vi "DT3120_NewDevice.vi"(8 "error in (no error)":errorcluster, 11 "Alias":string) -> (0 "error out":errorcluster, 1 "Frame Info":T1, 2 "CurDevCaps":T2, 3 "DevId":i32)   [LabVIEW 2013]
uses:
  olimg32.dll
  olfg32.dll
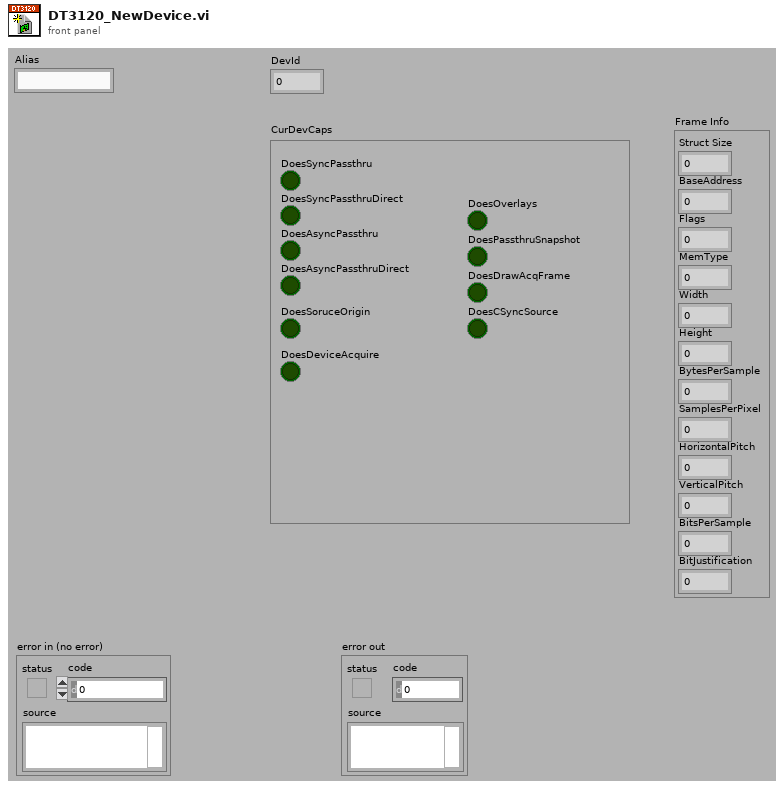
[diagram p1: front panel]
types:
  T1 = cluster{"Struct Size":u32, "BaseAddress":u32, "Flags":u32, "MemType":u32, "Width":u16, "Height":u16, "BytesPerSample":u16, "SamplesPerPixel":u16, "HorizontalPitch":u16, "VerticalPitch":u16, "BitsPerSample":u16, "BitJustification":u32}
  T2 = cluster{"DoesSyncPassthru":bool, "DoesSyncPassthruDirect":bool, "DoesAsyncPassthru":bool, "DoesAsyncPassthruDirect":bool, "DoesSoruceOrigin":bool, "DoesDeviceAcquire":bool, "DoesOverlays":bool, "DoesPassthruSnapshot":bool, "DoesDrawAcqFrame":bool, "DoesCSyncSource":bool}
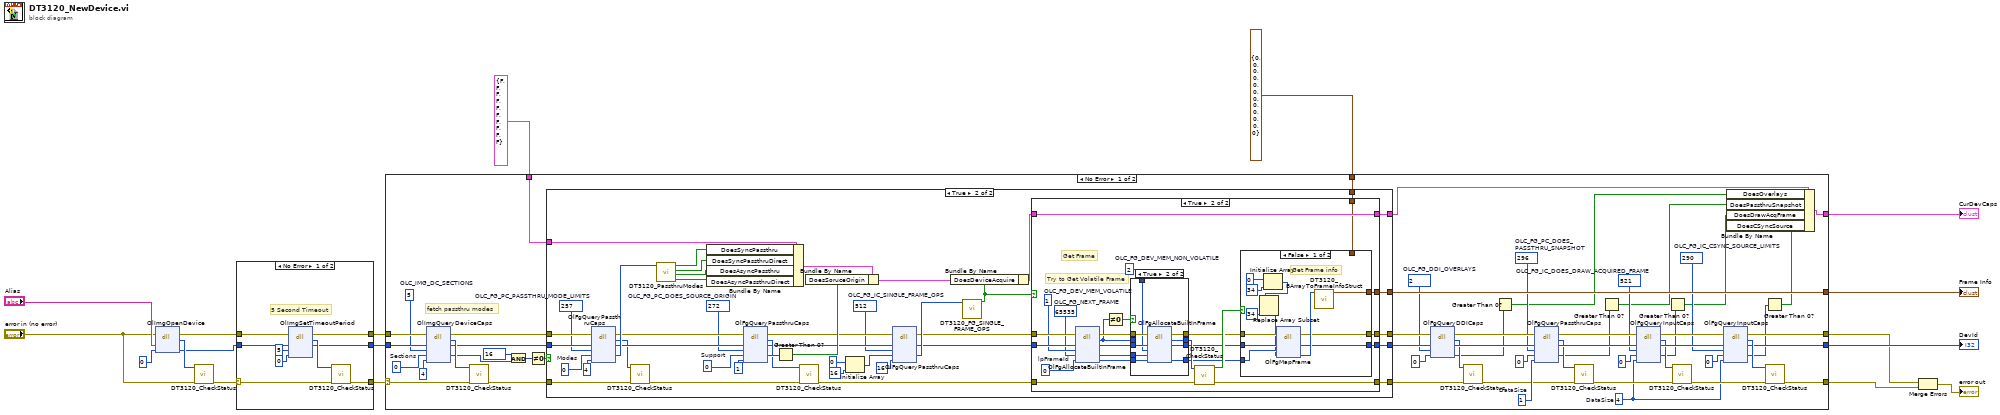
[diagram p0: block diagram]
diagram:
  n1 = dll-call lib="C:/Users/dhaehnel/Documents/Workspace/Labview_Workspace/labviewlib/MT Scan/SubVIs/olimg32.dll" fn="OlImgOpenDevice"(error in="error in (no error)", "Alias"="Alias", "lpDevId"=0 ("DevId")) -> (error out=w14:errorcluster, "Status"=w17:u32, "lpDevId"=w13:i32)  [unwired: 3 in, 1 out]
  n2 = call "DT3120_CheckStatus.vi"("error in"="error in (no error)", "Status"=w17) -> ("error out"=w12:errorcluster)  [unwired: 9 out]
  n3 = case shown="No Error" w12 {
    selector: w12 -> [w22 w30]
    tunnel: w14 -> [w27 w29]
    tunnel: w13 -> [w24 w28]
    tunnel: [w21 w29] -> w9
    tunnel: [w20 w30] -> w11
    tunnel: [w19 w28] -> w10
    frame No Error {
      # "5 Second Timeout"
      n4 = dll-call lib="C:/Users/dhaehnel/Documents/Workspace/Labview_Workspace/labviewlib/MT Scan/SubVIs/olimg32.dll" fn="OlImgSetTimeoutPeriod"(error in=w27, "DevId"=w24, "Period"=u32 5, "lpPeriod"=u32 0) -> (error out=w21:errorcluster, "Status"=w23:u32, "DevId"=w19:i32)  [unwired: 3 in, 2 out]
      n5 = call "DT3120_CheckStatus.vi"("error in"=w22, "Status"=w23) -> ("error out"=w20:errorcluster)  [unwired: 9 out]
    }
    frame Error {
    }
  }
  n6 = case shown="No Error" w11 {
    selector: w11 -> [w83 w196]
    tunnel: w9 -> [w86 w195]
    tunnel: w10 -> [w85 w194]
    tunnel: [w43 w195] -> w6
    tunnel: [w44 w196] -> w7
    tunnel: [w42 w194] -> w8
    tunnel: T2 {"DoesSyncPassthru"=FALSE, "DoesSyncPassthruDirect"=FALSE, "DoesAsyncPassthru"=FALSE, "DoesAsyncPassthruDirect"=FALSE, "DoesSoruceOrigin"=FALSE, "DoesDeviceAcquire"=FALSE, "DoesOverlays"=FALSE, "DoesPassthruSnapshot"=FALSE, "DoesDrawAcqFrame"=FALSE, "DoesCSyncSource"=FALSE} ("CurDevCaps") -> [w72 w193]
    tunnel: [w32 w193] -> w1
    tunnel: [w71 w192] -> w4
    tunnel: T1 {"Struct Size"=0, "BaseAddress"=0, "Flags"=0, "MemType"=0, "Width"=0, "Height"=0, "BytesPerSample"=0, "SamplesPerPixel"=0, "HorizontalPitch"=0, "VerticalPitch"=0, "BitsPerSample"=0, "BitJustification"=0} ("Frame Info") -> [w70 w192]
    frame No Error {
      w31 = u32 4  # DataSize
      w53 = 290  # OLC_FG_IC_CSYNC_SOURCE_LIMITS
      w60 = 521  # OLC_FG_IC_DOES_DRAW_ACQUIRED_FRAME
      w55 = u32 1  # DataSize
      w61 = 296  # OLC_FG_PC_DOES_PASSTHRU_SNAPSHOT
      w67 = 2  # OLC_FG_DDI_OVERLAYS
      w81 = u32 0  # Sections
      w82 = 5  # OLC_IMG_DC_SECTIONS
      # "fetch passthru modes"
      n7 = dll-call lib="C:/Users/dhaehnel/Documents/Workspace/Labview_Workspace/labviewlib/MT Scan/SubVIs/olimg32.dll" fn="OlImgQueryDeviceCaps"(error in=w86, "DevId"=w85, "Key"=w82, "lpData"=w81, "DataSize"=u32 4) -> (error out=w76:errorcluster, "Status"=w84:u32, "DevId"=w75:i32, "lpData"=w79:u32)  [unwired: 4 in, 1 out]
      n8 = call "DT3120_CheckStatus.vi"("error in"=w83, "Status"=w84) -> ("error out"=w74:errorcluster)  [unwired: 9 out]
      n9 = And(x=u32 16, y=w79) -> (x .and. y?=w77:u32)
      n10 = Not Equal To 0?(x=w77) -> (x != 0?=w73:bool)
      n11 = case shown="True" w73 {
        tunnel: w76 -> [w91 w134]
        tunnel: w75 -> [w90 w133]
        tunnel: w74 -> [w89 w122]
        tunnel: [w89 w101] -> w52
        tunnel: [w91 w97] -> w69
        tunnel: [w90 w96] -> w68
        tunnel: w72 -> [w88 w113]
        tunnel: [w88 w94] -> w33
        tunnel: [w87 w93] -> w71
        tunnel: w70 -> [w87 w92]
        frame False {
        }
        frame True {
          w125 = u8 0  # Support
          w109 = 512  # OLC_FG_IC_SINGLE_FRAME_OPS
          w126 = 272  # OLC_FG_PC_DOES_SOURCE_ORIGIN
          w131 = u32 0  # Modes
          w132 = 257  # OLC_FG_PC_PASSTHRU_MODE_LIMITS
          n12 = dll-call lib="C:/Users/dhaehnel/Documents/Workspace/Labview_Workspace/labviewlib/MT Scan/SubVIs/olfg32.dll" fn="OlFgQueryPassthruCaps"(error in=w134, "DevId"=w133, "Key"=w132, "lpData"=w131, "DataSize"=u32 4) -> (error out=w128:errorcluster, "Status"=w121:u32, "DevId"=w127:i32, "lpData"=w129:u32)  [unwired: 4 in, 1 out]
          n13 = call "DT3120_CheckStatus.vi"("error in"=w122, "Status"=w121) -> ("error out"=w120:errorcluster)  [unwired: 9 out]
          n14 = call "DT3120_PassthruModes.vi"("Modes"=w129) -> ("DoesAsyncPassthruDirect"=w114:bool, "DoesAsyncPassthru"=w115:bool, "DoesSyncPassthruDirect"=w116:bool, "DoesSyncPassthru"=w117:bool)  [unwired: 7 out]
          n15 = Bundle By Name(cluster=w113, "DoesSyncPassthru"=w117, "DoesSyncPassthruDirect"=w116, "DoesAsyncPassthru"=w115, "DoesAsyncPassthruDirect"=w114) -> (w112:T2)
          n16 = dll-call lib="C:/Users/dhaehnel/Documents/Workspace/Labview_Workspace/labviewlib/MT Scan/SubVIs/olfg32.dll" fn="OlFgQueryPassthruCaps"(error in=w128, "DevId"=w127, "Key"=w126, "lpData"=w125, "DataSize"=u32 1) -> (error out=w110:errorcluster, "Status"=w119:u32, "DevId"=w111:i32, "lpData"=w123:u8)  [unwired: 4 in, 1 out]
          n17 = Greater Than 0?(x=w123) -> (x > 0?=w118:bool)
          n18 = call "DT3120_CheckStatus.vi"("error in"=w120, "Status"=w119) -> ("error out"=w105:errorcluster)  [unwired: 9 out]
          n19 = Bundle By Name(cluster=w112, "DoesSoruceOrigin"=w118) -> (w106:T2)
          n20 = Initialize Array(u8 0, 16 ("dimension size")) -> (w99:u8[])
          n21 = dll-call lib="C:/Users/dhaehnel/Documents/Workspace/Labview_Workspace/labviewlib/MT Scan/SubVIs/olfg32.dll" fn="OlFgQueryPassthruCaps"(error in=w110, "DevId"=w111, "Key"=w109, "lpData"=w99, "DataSize"=u32 16) -> (error out=w103:errorcluster, "DevId"=w102:i32, "lpData"=w107:u8[])  [unwired: 4 in, 2 out]
          n22 = call "DT3120_FG_SINGLE_FRAME_OPS.vi"("OLT_FG_SINGLE_FRAME_OPS"=w107) -> ("DoesSyncPassthru"=w104:bool)  [unwired: 10 out]
          n23 = Bundle By Name(cluster=w106, "DoesDeviceAcquire"=w104) -> (w95:T2)
          n24 = case shown="True" w104 {
            tunnel: w105 -> [w139 w151]
            tunnel: w103 -> [w138 w163]
            tunnel: w102 -> [w137 w162]
            tunnel: [w139 w149] -> w101
            tunnel: [w138 w144] -> w97
            tunnel: [w137 w143] -> w96
            tunnel: w95 -> [w136 w142]
            tunnel: [w136 w142] -> w94
            tunnel: [w135 w141] -> w93
            tunnel: w92 -> [w135 w140]
            frame False {
            }
            frame True {
              w160 = u16 65535  # OLC_FG_NEXT_FRAME
              w153 = 2  # OLC_FG_DEV_MEM_NON_VOLATILE
              w155 = u32 0  # lpFrameId
              w161 = 1  # OLC_FG_DEV_MEM_VOLATILE
              # "Try to Get Volatile Frame"
              # "Get Frame"
              n25 = dll-call lib="C:/Users/dhaehnel/Documents/Workspace/Labview_Workspace/labviewlib/MT Scan/SubVIs/olfg32.dll" fn="OlFgAllocateBuiltInFrame"(error in=w163, "DevId"=w162, "MemType"=w161, "BufNum"=w160, "lpFrameId"=w155) -> (error out=w158:errorcluster, "Status"=w152:u32, "DevId"=w157:i32, "BufNum"=w156:u16, "lpFrameId"=w154:u32)  [unwired: 3 in, 1 out]
              n26 = Not Equal To 0?(x=w152) -> (x != 0?=w159:bool)
              n27 = case shown="True" w159 {
                tunnel: w158 -> [w182 w191]
                tunnel: w157 -> [w181 w190]
                tunnel: w156 -> [_ w189]
                tunnel: w154 -> [w180 w188]
                tunnel: w153 -> [_ w187]
                tunnel: [w182 w186] -> w147
                tunnel: [w181 w185] -> w146
                tunnel: [w180 w184] -> w145
                tunnel: w152 -> [w179 _]
                tunnel: [w179 w183] -> w150
                frame False {
                }
                frame True {
                  n28 = dll-call lib="C:/Users/dhaehnel/Documents/Workspace/Labview_Workspace/labviewlib/MT Scan/SubVIs/olfg32.dll" fn="OlFgAllocateBuiltInFrame"(error in=w191, "DevId"=w190, "MemType"=w187, "BufNum"=w189, "lpFrameId"=w188) -> (error out=w186:errorcluster, "Status"=w183:u32, "DevId"=w185:i32, "lpFrameId"=w184:u32)  [unwired: 4 in, 1 out]
                }
              }
              n29 = call "DT3120_CheckStatus.vi"("error in"=w151, "Status"=w150) -> ("error out"=w149:errorcluster, "New Error?"=w148:bool)  [unwired: 8 out]
              n30 = case shown="False" w148 {
                tunnel: w147 -> [w175 w178]
                tunnel: w146 -> [w174 w177]
                tunnel: w145 -> [w173 _]
                tunnel: [w166 w178] -> w144
                tunnel: [w165 w177] -> w143
                tunnel: [w164 w176] -> w141
                tunnel: w140 -> [_ w176]
                frame False {
                  # "Get Frame info"
                  n31 = Initialize Array(u8 0, 34 ("dimension size")) -> (w171:u8[])
                  n32 = Replace Array Subset(array=w171, new element=u8 34 ("dimension size")) -> (w168:u8[])  [unwired: 1 in]
                  n33 = dll-call lib="C:/Users/dhaehnel/Documents/Workspace/Labview_Workspace/labviewlib/MT Scan/SubVIs/olfg32.dll" fn="OlFgMapFrame"(error in=w175, "DevId"=w174, "FrameID"=w173, "lpFrameInfo"=w168) -> (error out=w166:errorcluster, "DevId"=w165:i32, "lpFrameInfo"=w167:u8[])  [unwired: 3 in, 2 out]
                  n34 = call "DT3120_BArrayToFrameInfoStruct.vi"("lpFrameInfo"=w167) -> ("Frame Info"=w164:T1)  [unwired: 10 out]
                }
                frame True {
                }
              }
            }
          }
        }
      }
      n35 = dll-call lib="C:/Users/dhaehnel/Documents/Workspace/Labview_Workspace/labviewlib/MT Scan/SubVIs/olfg32.dll" fn="OlFgQueryDDICaps"(error in=w69, "DevId"=w68, "Key"=w67, "lpBool"=u8 0) -> (error out=w65:errorcluster, "Status"=w51:u32, "DevId"=w63:i32, "lpBool"=w41:u8)  [unwired: 3 in, 1 out]
      n36 = call "DT3120_CheckStatus.vi"("error in"=w52, "Status"=w51) -> ("error out"=w50:errorcluster)  [unwired: 9 out]
      n37 = Greater Than 0?(x=w41) -> (x > 0?=w34:bool)
      n38 = dll-call lib="C:/Users/dhaehnel/Documents/Workspace/Labview_Workspace/labviewlib/MT Scan/SubVIs/olfg32.dll" fn="OlFgQueryPassthruCaps"(error in=w65, "DevId"=w63, "Key"=w61, "lpData"=u8 0, "DataSize"=w55) -> (error out=w64:errorcluster, "Status"=w47:u32, "DevId"=w62:i32, "lpData"=w40:u8)  [unwired: 4 in, 1 out]
      n39 = call "DT3120_CheckStatus.vi"("error in"=w50, "Status"=w47) -> ("error out"=w49:errorcluster)  [unwired: 9 out]
      n40 = Greater Than 0?(x=w40) -> (x > 0?=w35:bool)
      n41 = dll-call lib="C:/Users/dhaehnel/Documents/Workspace/Labview_Workspace/labviewlib/MT Scan/SubVIs/olfg32.dll" fn="OlFgQueryInputCaps"(error in=w64, "DevId"=w62, "Key"=w60, "lpData"=u32 0, "DataSize"=w31) -> (error out=w56:errorcluster, "Status"=w46:u32, "DevId"=w54:i32, "lpData"=w39:u32)  [unwired: 4 in, 1 out]
      n42 = Greater Than 0?(x=w39) -> (x > 0?=w36:bool)
      n43 = call "DT3120_CheckStatus.vi"("error in"=w49, "Status"=w46) -> ("error out"=w48:errorcluster)  [unwired: 9 out]
      n44 = dll-call lib="C:/Users/dhaehnel/Documents/Workspace/Labview_Workspace/labviewlib/MT Scan/SubVIs/olfg32.dll" fn="OlFgQueryInputCaps"(error in=w56, "DevId"=w54, "Key"=w53, "lpData"=u32 0, "DataSize"=w31) -> (error out=w43:errorcluster, "Status"=w45:u32, "DevId"=w42:i32, "lpData"=w38:u32)  [unwired: 4 in, 1 out]
      n45 = Greater Than 0?(x=w38) -> (x > 0?=w37:bool)
      n46 = Bundle By Name(cluster=w33, "DoesOverlays"=w34, "DoesPassthruSnapshot"=w35, "DoesDrawAcqFrame"=w36, "DoesCSyncSource"=w37) -> (w32:T2)
      n47 = call "DT3120_CheckStatus.vi"("error in"=w48, "Status"=w45) -> ("error out"=w44:errorcluster)  [unwired: 9 out]
    }
    frame Error {
    }
  }
  "CurDevCaps" <- w1
  "DevId" <- w8
  "Frame Info" <- w4
  n48 = Merge Errors(w6, w7) -> (→"error out":errorcluster)
